vi "TB-Create Stimulus.vi"(0 "state":T1, 9 "Num":i32, 11 "error in (no error)":errorcluster, 12 "Fine adjust (dB)":dbl) -> (4 "state out":T1, 8 "Stimulus":dbl[][](array[numeric]), 15 "error out":errorcluster)   [LabVIEW 2020]
uses:
  Typedefs/TB-Stimulus State.ctl
  epl-vi-lib/Signal Synthesis VIs/4th Generation/Classes/SignalManager/SignalManager.lvclass
  <vilib>/sound2/lvsound2.llb/Sound File Refnum.ctl
  4dce84e5-d5b4-4a54-8c7d-6deba4adc8d9.vi
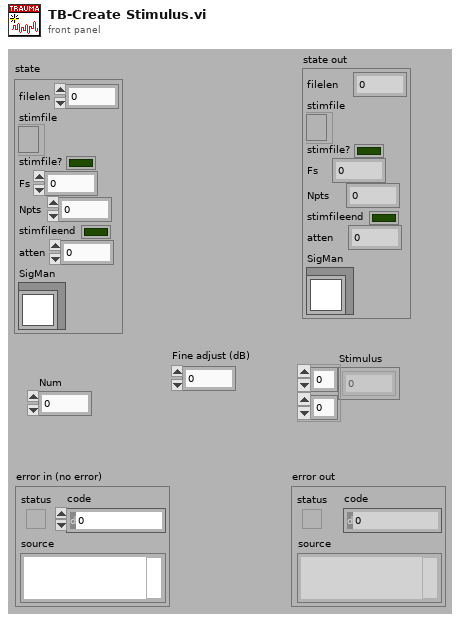
[diagram p1: front panel]
types:
  T1 = typedef "TB-Stimulus State.ctl" = cluster{"filelen":i32, "stimfile":T2, "stimfile?":bool, "Fs":dbl, "Npts":i32, "stimfileend":bool, "atten":dbl, "SigMan":refnum<class "SignalManager.lvclass">}
  T2 = typedef "Sound File Refnum.ctl" = refnum<file>
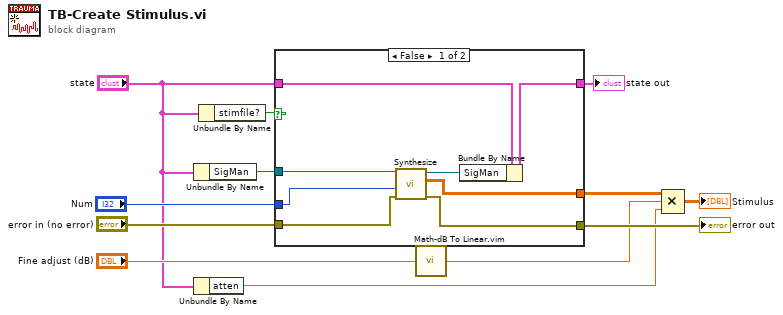
[diagram p0: block diagram]
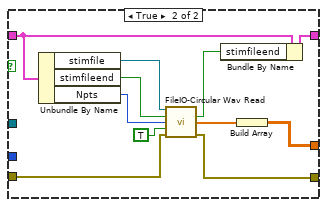
[diagram p2: hidden frame]
diagram:
  n1 = Unbundle By Name("state") -> ("SigMan"=w1:refnum<class "SignalManager.lvclass">)
  n2 = Unbundle By Name("state") -> ("atten"=w5:dbl)
  n3 = Unbundle By Name("state") -> ("stimfile?"=w7:bool)
  n4 = case shown="False" w7 {
    tunnel: "error in (no error)" -> [w18 w25]
    tunnel: w1 -> [w19 _]
    tunnel: [w15 w21] -> w3
    tunnel: [w16 w24] -> w11
    tunnel: "state" -> [w20 w31]
    tunnel: [w14 w30] -> w6
    tunnel: "Num" -> [w17 _]
    frame False {
      n5 = call "Synthesize.vi"("error in (no error)"=w18, "Repetition"=w17, "SigMan in"=w19) -> ("error out"=w16:errorcluster, "Array"=w15:dbl[][], "SigMan out"=w13:refnum<class "SignalManager.lvclass">)  [unwired: 6 in]
      n6 = Bundle By Name(cluster=w20, "SigMan"=w13) -> (w14:T1)
    }
    frame True {
      n7 = Unbundle By Name(w31) -> ("stimfile"=w28:T2, "stimfileend"=w27:bool, "Npts"=w29:i32)
      n8 = call "FileIO-Circular Wav Read.vi"("Fileref in"=w28, "stimfileend"=w27, "Nread"=w29, "Loop?"=TRUE, "error in (no error)"=w25) -> ("end of file?"=w22:bool, "Y"=w23:dbl[], "error out"=w24:errorcluster)  [unwired: 6 in, 2 out]
      n9 = Bundle By Name(cluster=w31, "stimfileend"=w22) -> (w30:T1)
      n10 = Build Array(w23) -> (w21:dbl[][])
    }
  }
  "error out" <- w11
  "state out" <- w6
  n11 = call "Math-dB To Linear.vim"("dB"="Fine adjust (dB)") -> ("linear"=w8:dbl)
  n12 = Compound Arithmetic op=MULTIPLY(w3, w8, w5) -> (→"Stimulus":dbl[][])
